vi "Running Total.vi"(11 "Numeric 4":dbl) -> (3 "String":string)   [LabVIEW 2020]
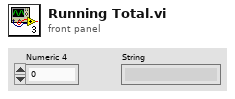
[diagram p1: front panel]
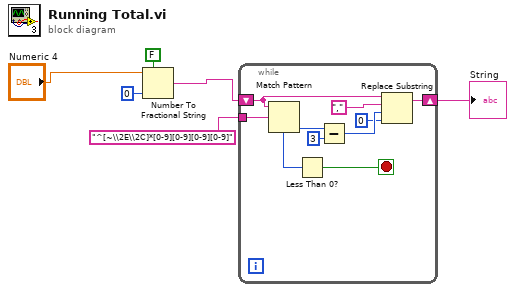
[diagram p0: block diagram]
diagram:
  n1 = Number To Fractional String(use system decimal point (T)=FALSE, number="Numeric 4", precision (6)=i16 0) -> (F-format string=w3:string)  [unwired: 1 in]
  n2 = while {
    shift-right: [w13] -> w2
    shift-left: w3 -> [w8]
    tunnel: "^[~\\2E\\2C]*[0-9][0-9][0-9][0-9]" ("regular expression") -> [w11]
    stop <- w15 stop-if-true
    n3 = Match Pattern(string=w8, regular expression=w11) -> (offset past match=w7:i32)  [unwired: 1 in, 3 out]
    n4 = Less Than 0?(x=w7) -> (x < 0?=w15:bool)
    n5 = Subtract(x=w7, y=3) -> (x-y=w10:i32)
    n6 = Replace Substring(2:0 ("length (len. of substring)"), 3:w10, 4:"," ("substring (\"\")"), 5:w8) -> (1:w13:string)  [unwired: 1 out]
  }
  "String" <- w2
